vi "Keyence LJ-V7000 Read Measurement Data.vi"() -> ()   [LabVIEW 2014]
doc: "This example mainly indicates how to acquire measurement results from controllers by using <B>Read Measurement Data</B> VI.\n\n<B>Note</B>:\nIf you execute this example, set the operation mode of the controller to the advanced mode."
uses:
  Public/constant/Comm Interface.ctl
  Public/Clusters/Ethernet Config.ctl
  Public/constant/Measure Data Info.ctl
  Public/constant/Judge Result.ctl
  Keyence LJ-V7000.lvlib
panel:
  in  "Stop VI":bool
  out "Measure Data":T3(array[cluster]) {"Judge Result" items=["HI"=1, "GO"=2, "LO"=4, "ALARM"=5]; "Data Info" items=["VALID", "ALARM", "WAIT"]}
  in  "Ethernet Config":T4={"IP Address"=[192, 168, 0, 1], "Port No"=24691}
  in  "Comm Interface":T5
  # "Communication Configuration"
  # "Output from Read Measurement Data VI"
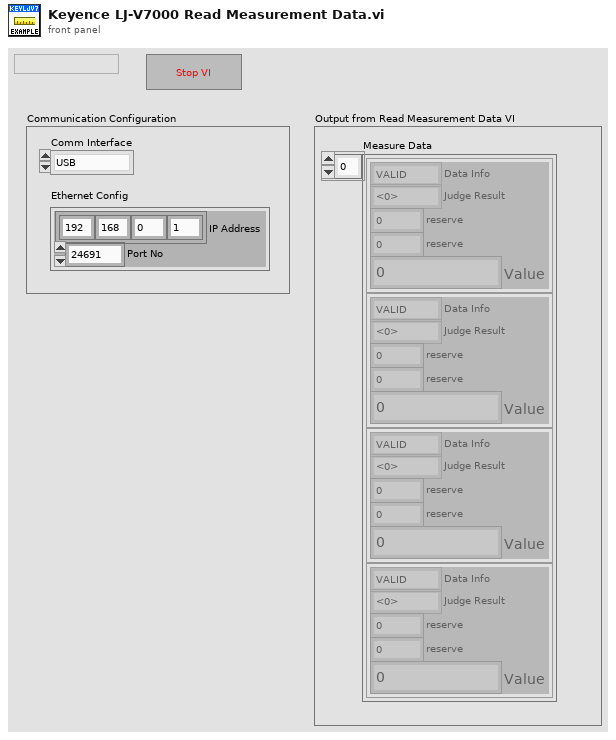
[diagram p1: front panel]
types:
  T1 = typedef "Keyence LJ-V7000.lvlib/Measure Data Info.ctl" = u8
  T2 = typedef "Keyence LJ-V7000.lvlib/Judge Result.ctl" = u8
  T3 = cluster{"Data Info":T1, "Judge Result":T2, "reserve":u8, "reserve":u8, "Value":sgl}[]
  T4 = typedef "Keyence LJ-V7000.lvlib/Ethernet Config.ctl" = cluster{"IP Address":u8[], "Port No":u16}
  T5 = typedef "Keyence LJ-V7000.lvlib/Comm Interface.ctl" = enum8{"USB", "ETHERNET"}
  T6 = typedef "Keyence LJ-V7000.lvlib/Measure Data.ctl" = cluster{"Data Info":T1, "Judge Result":T2, "reserve":u8, "reserve":u8, "Value":sgl}
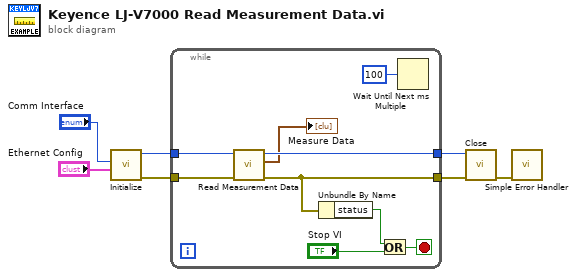
[diagram p0: block diagram]
diagram:
  n1 = call "Initialize.vi"("Ethernet Config"="Ethernet Config", "Comm Interface"="Comm Interface") -> ("error out"=w7:errorcluster, "Device ID out"=w6:i32)  [unwired: 8 in]
  n2 = while {
    tunnel: w7 -> [w16]
    tunnel: w6 -> [w15]
    tunnel: [w11] -> w5
    tunnel: [w14] -> w4
    stop <- w8 stop-if-true
    n3 = call "Read Measurement Data.vi"("error in (no error)"=w16, "Device ID (0)"=w15) -> ("error out"=w11:errorcluster, "Measure Data"=→"Measure Data":T6[], "Device ID out"=w14:i32)  [unwired: 7 in]
    n4 = Unbundle By Name(w11) -> ("status"=w9:bool)
    n5 = Or(x=w9, y="Stop VI") -> (x .or. y?=w8:bool)
    n6 = Wait Until Next ms Multiple(millisecond multiple=u32 100 ("ミリ秒倍数")) -> ()  [unwired: 1 out]
  }
  n7 = call "Close.vi"("error in (no error)"=w5, "Device ID (0)"=w4) -> ("error out"=w1:errorcluster)  [unwired: 8 in, 1 out]
  n8 = call <vilib>:"Simple Error Handler.vi"("error in (no error)"=w1) -> ()  [unwired: 4 in, 5 out]
